vi "Result_Test.vi"(8 "error in (no error)":errorcluster caption="entrée d'erreur (pas d'erreur)", 11 "Get_Voltage en entrée":refnum<class "Read_Multimeter.lvclass">) -> (0 "error out":errorcluster caption="sortie d'erreur", 3 "Get_Voltage en sortie":refnum<class "Read_Multimeter.lvclass">)   [LabVIEW 2020, in "Library Test.lvlib" / "Read_Multimeter.lvclass"]
uses:
  Read_Multimeter.lvclass
  C:/Users/ngarcin/OneDrive - Altyor/Standard TB/Class/Test/Test (Default)/Test (Default).lvclass
  Test_Wtih_Instr/Test_With_Inst.lvclass
  Read_Multimeter.lvclass/Read_Multimeter.ctl
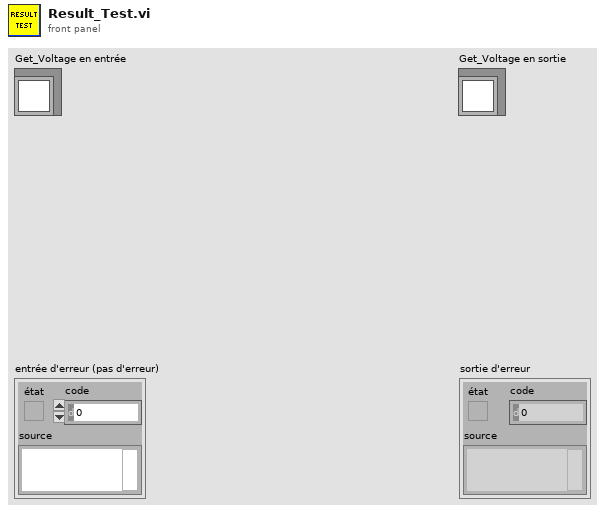
[diagram p1: front panel]
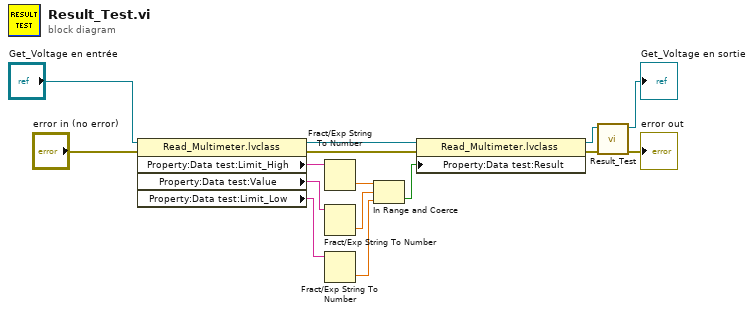
[diagram p0: block diagram]
diagram:
  n1 = property class="Read_Multimeter.lvclass"(reference="Get_Voltage en entrée", error in="error in (no error)") -> (reference out=w6:refnum<class "Read_Multimeter.lvclass">, error out=w5:errorcluster, "Property:Data test:Limit_High"=w12:string, "Property:Data test:Value"=w10:string, "Property:Data test:Limit_Low"=w11:string)
  n2 = Fract/Exp String To Number(string=w12) -> (number=w9:dbl)  [unwired: 3 in, 1 out]
  n3 = Fract/Exp String To Number(string=w10) -> (number=w8:dbl)  [unwired: 3 in, 1 out]
  n4 = Fract/Exp String To Number(string=w11) -> (number=w7:dbl)  [unwired: 3 in, 1 out]
  n5 = In Range and Coerce(upper limit=w9, x=w8, lower limit=w7) -> (In Range?=w4:bool)  [unwired: 1 out]
  n6 = property class="Read_Multimeter.lvclass"(reference=w6, error in=w5, "Property:Data test:Result"=w4) -> (reference out=w2:refnum<class "Read_Multimeter.lvclass">, error out=w3:errorcluster)
  n7 = call-parent "Result_Test.vi"("error in (no error)"=w3, "Test_With_Inst en entrée"=w2) -> ("error out"=→"error out":errorcluster, "Test_With_Inst en sortie"=→"Get_Voltage en sortie":refnum<class "Read_Multimeter.lvclass">)  [unwired: 8 in]
